vi "Get JSON Config.vi"(8 "error in (no error)":errorcluster, 11 "CFG Base in":refnum<class "CFG Base.lvclass">) -> (0 "error out":errorcluster, 2 "<JSON>Config>":string, 3 "CFG Base out":refnum<class "CFG Base.lvclass">)   [LabVIEW 2023, in "HAL GOOP4.lvlib" / "CFG Base.lvclass"]
uses:
  CFG Base.lvclass
  CFG Base.lvclass/CFG Base.ctl
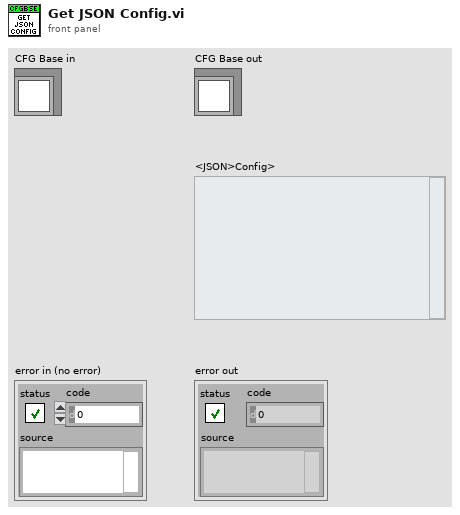
[diagram p1: front panel]
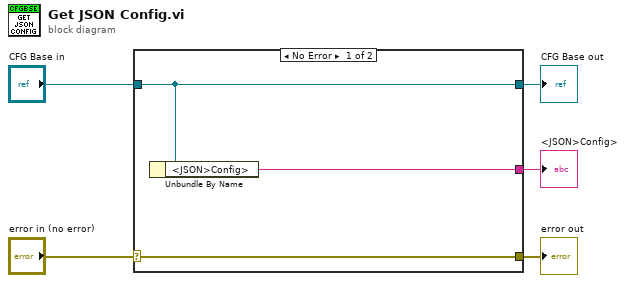
[diagram p0: block diagram]
diagram:
  n1 = case shown="No Error" "error in (no error)" {
    selector: "error in (no error)" -> [w8 w9]
    tunnel: [w8 w9] -> w4
    tunnel: [w7 w10] -> w2
    tunnel: "CFG Base in" -> [w7 w10]
    tunnel: [w6 _] -> w1
    frame No Error {
      n2 = Unbundle By Name(w7) -> ("<JSON>Config>"=w6:string)
    }
    frame Error {
    }
  }
  "error out" <- w4
  "CFG Base out" <- w2
  "<JSON>Config>" <- w1
